vi "Message Send.vi"(0 "Message":string, 1 "Destination":string) -> ()   [LabVIEW 2009]
doc: "This is the general purpose VI to send messages. It takes two inputs: the destination and the message.\n\nIf the destination does not exist (seom VI created but not added to the list on the diagram) then only the 0th frame in the case sequences is executed and nothing is done.\n\nIf the destination does exist then the new message is added to the list of existing messages for that destination. Finally the occurence for that destinator is set so that anyone wating for the occurence can stop waiting."
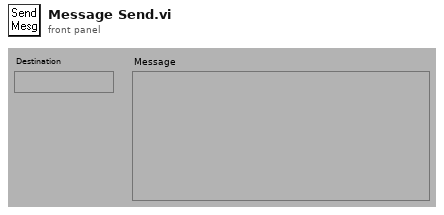
[diagram p1: front panel]
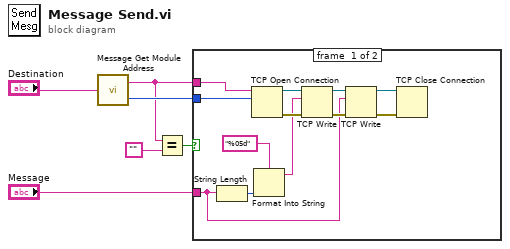
[diagram p0: block diagram]
diagram:
  n1 = call "Message Get Module Address.vi"("Module"="Destination") -> ("Address"=w3:string, "Port"=w6:u16)
  n2 = Equal?(x=w3, y="") -> (x = y?=w1:bool)
  n3 = case shown="False" w1 {
    tunnel: w3 -> [w18 _]
    tunnel: w6 -> [w17 _]
    tunnel: "Message" -> [w7 _]
    frame #0 {
      n4 = String Length(string=w7) -> (length=w9:i32)
      n5 = TCP Open Connection(address=w18, remote port or service name=w17) -> (connection ID=w11:refnum<k5>, error out=w12:errorcluster)  [unwired: 3 in]
      n6 = Format Into String(format string="%05d" ("Format String"), w9) -> (resulting string=w10:string)  [unwired: 2 in, 1 out]
      n7 = TCP Write(connection ID=w11, data in=w10, error in (no error)=w12) -> (connection ID out=w14:refnum<k5>, error out=w13:errorcluster)  [unwired: 1 in, 1 out]
      n8 = TCP Write(connection ID=w14, data in=w7, error in (no error)=w13) -> (connection ID out=w16:refnum<k5>, error out=w15:errorcluster)  [unwired: 1 in, 1 out]
      n9 = TCP Close Connection(connection ID=w16, error in (no error)=w15) -> ()  [unwired: 1 in, 2 out]
    }
    frame #1 {
    }
  }
